vi "Anritsu VNA Initialize.vi"(8 "error in (no error)":errorcluster, 11 "Configuration":T2={"BusType"=enum."GPIB", "GPIB Bus"=0, "GPIB Address"=6, "IP"=0, "COM"=1, "Baud Rate"=enum."9600", "USB Device"=0, "Instrument S\\N"="", "SCIL Address"=16} {"USB Device" max=31 step=1}) -> (0 "error out":errorcluster {"code" format="%.0x"}, 3 "dup VISA Resource Name":refnum<visa-resource-name>, 5 "Anritsu VNA":T1)   [LabVIEW 2011]
uses:
  VNA Configuration.ctl
  TypeDefs/Anritsu VNA Instrument Info.ctl
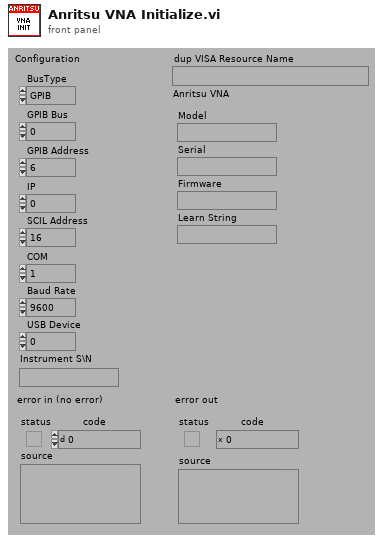
[diagram p1: front panel]
types:
  T1 = typedef "Anritsu VNA Instrument Info.ctl" = cluster{"Model":string, "Serial":string, "Firmware":string, "Learn String":string}
  T2 = typedef "VNA Configuration.ctl" = cluster{"BusType":enum32{"GPIB", "LAN/IP", "Serial", "USB"}, "GPIB Bus":i32, "GPIB Address":i32, "IP":u32, "COM":i32, "Baud Rate":enum32{"300", "600", "1200", "2400", "4800", "9600"}, "USB Device":u32, "Instrument S\\N":string, "SCIL Address":i32}
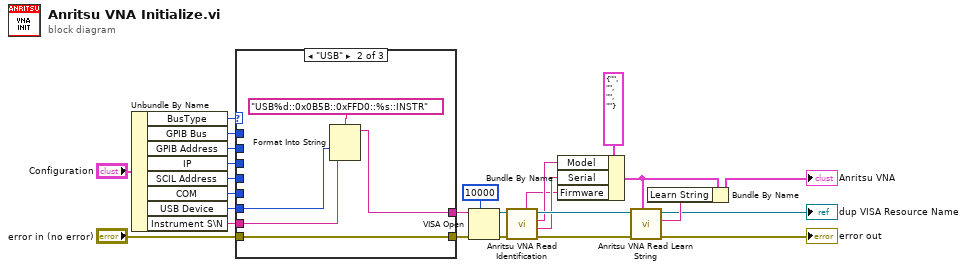
[diagram p0: block diagram]
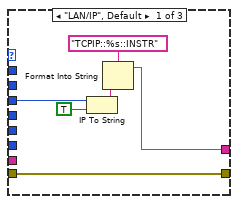
[diagram p2: hidden frame]
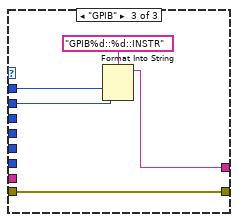
[diagram p3: hidden frame]
diagram:
  n1 = Unbundle By Name("Configuration") -> ("BusType"=w25:enum32{"GPIB", "LAN/IP", "Serial", "USB"}, "GPIB Bus"=w24:i32, "GPIB Address"=w23:i32, "IP"=w20:u32, "SCIL Address"=w1:i32, "COM"=w22:i32, "USB Device"=w19:u32, "Instrument S\\N"=w3:string)
  n2 = case shown="\"USB\"" w25 {
    tunnel: "error in (no error)" -> [w28 w35 w41]
    tunnel: w24 -> [_ _ w40]
    tunnel: w23 -> [_ _ w39]
    tunnel: [w27 w34 w38] -> w2
    tunnel: [w28 w35 w41] -> w7
    tunnel: w22 -> [_ _ _]
    tunnel: w20 -> [w29 _ _]
    tunnel: w19 -> [_ w36 _]
    tunnel: w3 -> [_ w33 _]
    tunnel: w1 -> [_ _ _]
    frame "LAN/IP", Default {
      n3 = IP To String(1:TRUE ("dot notation? (F)"), 2:w29) -> (0:w31:string)
      n4 = Format Into String(format string="TCPIP::%s::INSTR", w31) -> (resulting string=w27:string)  [unwired: 2 in, 1 out]
    }
    frame "USB" {
      n5 = Format Into String(format string="USB%d::0x0B5B::0xFFD0::%s::INSTR", w36, w33) -> (resulting string=w34:string)  [unwired: 2 in, 1 out]
    }
    frame "GPIB" {
      n6 = Format Into String(format string="GPIB%d::%d::INSTR", w40, w39) -> (resulting string=w38:string)  [unwired: 2 in, 1 out]
    }
  }
  n7 = VISA Open(timeout (0)=u32 10000 ("VISA Open timeout (0)"), error in (no error)=w7, VISA resource name=w2) -> (VISA resource name=w17:refnum<visa-resource-name>, error out=w18:errorcluster)  [unwired: 2 out]
  n8 = call "Anritsu VNA Read Identification.vi"("error in (no error)"=w18, "VISA Resource Name"=w17) -> ("error out"=w14:errorcluster, "Serial Number"=w12:string, "Model Number"=w11:string, "dup VISA Resource Name"=w13:refnum<visa-resource-name>, "Firmware"=w10:string)  [unwired: 5 out]
  n9 = Bundle By Name(cluster=T1 {"Model"="", "Serial"="", "Firmware"="", "Learn String"=""} ("Anritsu VNA"), "Model"=w11, "Serial"=w12, "Firmware"=w10) -> (w15:T1)
  n10 = call "Anritsu VNA Read Learn String.vi"("Anritsu VNA"=w15, "error in (no error)"=w14, "VISA Resource Name"=w13) -> ("error out"=→"error out":errorcluster, "Learn String"=w16:string, "dup VISA Resource Name"=→"dup VISA Resource Name":refnum<visa-resource-name>)  [unwired: 6 out]
  n11 = Bundle By Name(cluster=w15, "Learn String"=w16) -> (→"Anritsu VNA":T1)
